vi "Parse Next Template.vi"(9 "Text":string, 11 "Locals in":refnum<class "Value Tree.lvclass">) -> (1 "Remaining":string, 2 "Value Name":string, 3 "Namespace":string, 5 "Locals":refnum<class "Value Tree.lvclass">, 7 "Before":string)   [LabVIEW 2020, in "HTTP Server.lvlib" / "BasicTemplater.lvclass"]
uses:
  BasicTemplater.lvclass
  Value Tree/Value Tree.lvclass
  Value Tree/Value Tree.lvclass/Value Tree.ctl
  Value Tree/Add Local.vi
  BasicTemplater.lvclass/BasicTemplater.ctl
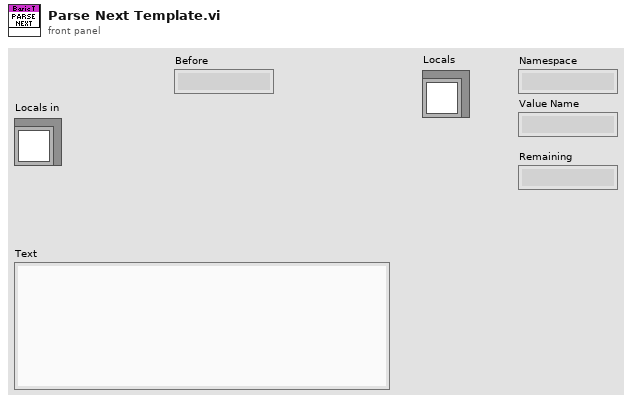
[diagram p1: front panel]
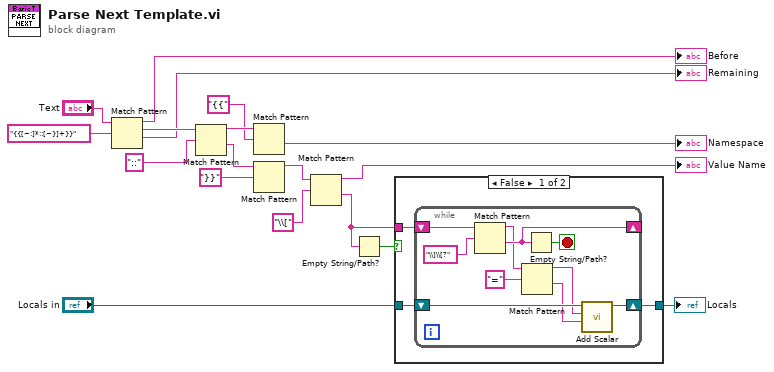
[diagram p0: block diagram]
diagram:
  n1 = Match Pattern(string="Text", regular expression="{{[~:]*::[~}]+}}") -> (before substring=→"Before":string, match substring=w16:string, after substring=→"Remaining":string)  [unwired: 1 in, 1 out]
  n2 = Match Pattern(string=w16, regular expression="::") -> (before substring=w14:string, after substring=w12:string)  [unwired: 1 in, 2 out]
  n3 = Match Pattern(string=w14, regular expression="{{") -> (after substring=→"Namespace":string)  [unwired: 1 in, 3 out]
  n4 = Match Pattern(string=w12, regular expression="}}") -> (before substring=w7:string)  [unwired: 1 in, 3 out]
  n5 = Match Pattern(string=w7, regular expression="\\[") -> (before substring=→"Value Name":string, after substring=w4:string)  [unwired: 1 in, 2 out]
  n6 = Empty String/Path?(string/path=w4) -> (empty?=w3:bool)
  n7 = case shown="False" w3 {
    tunnel: "Locals in" -> [w21 w32]
    tunnel: [w20 w32] -> w5
    tunnel: w4 -> [w19 _]
    frame False {
      n8 = while {
        shift-right: [w29] -> _
        shift-left: w19 -> [w31]
        shift-right: [w22] -> w20
        shift-left: w21 -> [w25]
        stop <- w28 stop-if-true
        n9 = Match Pattern(string=w31, regular expression="\\]\\[?") -> (before substring=w27:string, after substring=w29:string)  [unwired: 1 in, 2 out]
        n10 = Match Pattern(string=w27, regular expression="=") -> (before substring=w24:string, after substring=w23:string)  [unwired: 1 in, 2 out]
        n11 = Empty String/Path?(string/path=w29) -> (empty?=w28:bool)
        n12 = call "Add Scalar.vi"("Value"=w23, "Name"=w24, "TemplateLocals in"=w25) -> ("TemplateLocals out"=w22:refnum<class "Value Tree.lvclass">)  [unwired: 6 in, 2 out]
      }
    }
    frame True {
    }
  }
  "Locals" <- w5
